vi "NET control example with SP and WFM channels.vi"(8 "error in (no error)":errorcluster, 11 "Node Ptr":T1 format="%.0x") -> (0 "error out":errorcluster)   [LabVIEW 2015]
uses:
  <vilib>/NI Veristand/Custom Device API/Custom Device Item Ref.ctl
  NationalInstruments.VeriStand.SystemStorageUI
  NationalInstruments.VeriStand.SystemStorage
  <vilib>/NI Veristand/Custom Device API/Get Item Property (Dependent Node Pointer).vi
  Shared/Globals/Global GUIDs.vi
  <vilib>/NI Veristand/Custom Device Tools/Custom Device Utility Library/NI VeriStand - Search for All Items by GUID.vi
  <vilib>/NI Veristand/Custom Device API/Set Item Property (Dependent Node Pointer).vi
  <vilib>/NI VeriStand/Custom Device API/Custom Device API.lvlib
  System Explorer/Waveform Data Logger System Explorer.lvlib
  <vilib>/NI VeriStand/Custom Device Tools/Custom Device Utility Library/Custom Device Utility Library.lvlib
  Shared/Waveform Data Logger Shared.lvlib
  <vilib>/NI VeriStand/UI Controls/Single Node Browser/NI_VS UI Single Node Browser.lvlib
panel:
  out ".not. x?":bool
  in  "Source Waveform":refnum<k24>(container)
  in  "Header 2":cluster{"Section Name":string}={"Section Name"="TDMS Data Log Files"}
  in  "Remove":bool
  in  "TDMS Log Files":i32(listbox)
  in  "Add File":bool
  in  "Header":cluster{"Section Name":string}={"Section Name"="Waveform Data Logger Settings"}
  in  "Name":string
  # "TODO: Waveform queue size (auto 3x # wfms, or manual)"
  # "TODO: Mode: one log at a time, one active trigger per log, or log every trigger\n-don't do this. instead using logging group, and allow multiple concurrent triggers for logs with stop trig of \"Duration\""
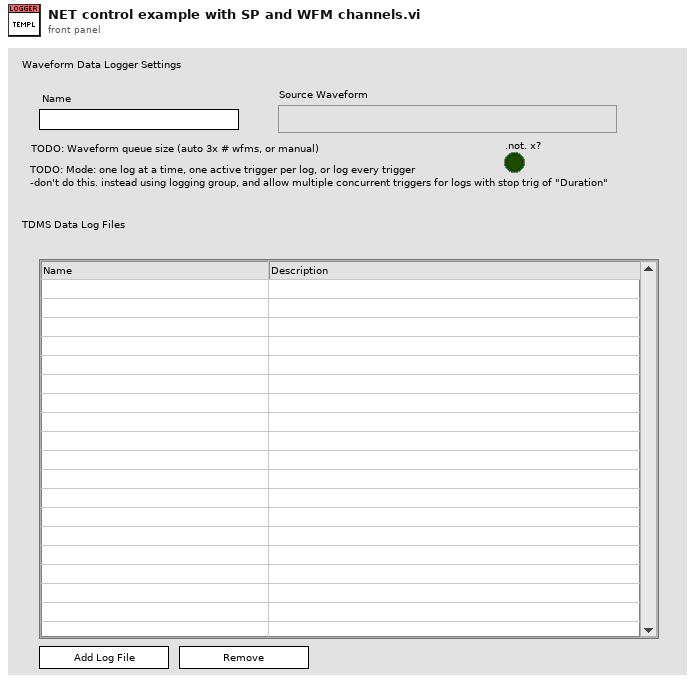
[diagram p1: front panel]
types:
  T1 = typedef "Custom Device API.lvlib/Custom Device Item Ref.ctl" = u64
  T2 = typedef "Custom Device API.lvlib/Custom Device Item Info.ctl" = cluster{"Name":string, "Is Channel":bool, "GUID":string, "Is Waveform":bool}
  T3 = typedef "Custom Device API.lvlib/Custom Device Pointer.ctl" = refnum<k24>
  T4 = typedef "NI_VS UI Single Node Browser.lvlib/Callback Type.ctl" = cluster{"Net Callbacks":refnum<k27>[], "Event":refnum<user-event>}
  T5 = typedef "Custom Device API.lvlib/Custom Device Commands.ctl" = enum16{"Default", "Item renamed", "Shutdown", "Dynamic button pressed"}
  T6 = typedef "LVRowAndColumnTypeDef.ctl" = cluster{"Row":i32, "Column":i32}
  T7 = typedef "NI_VS UI Single Node Browser.lvlib/Node Ref.ctl" = refnum<k24>
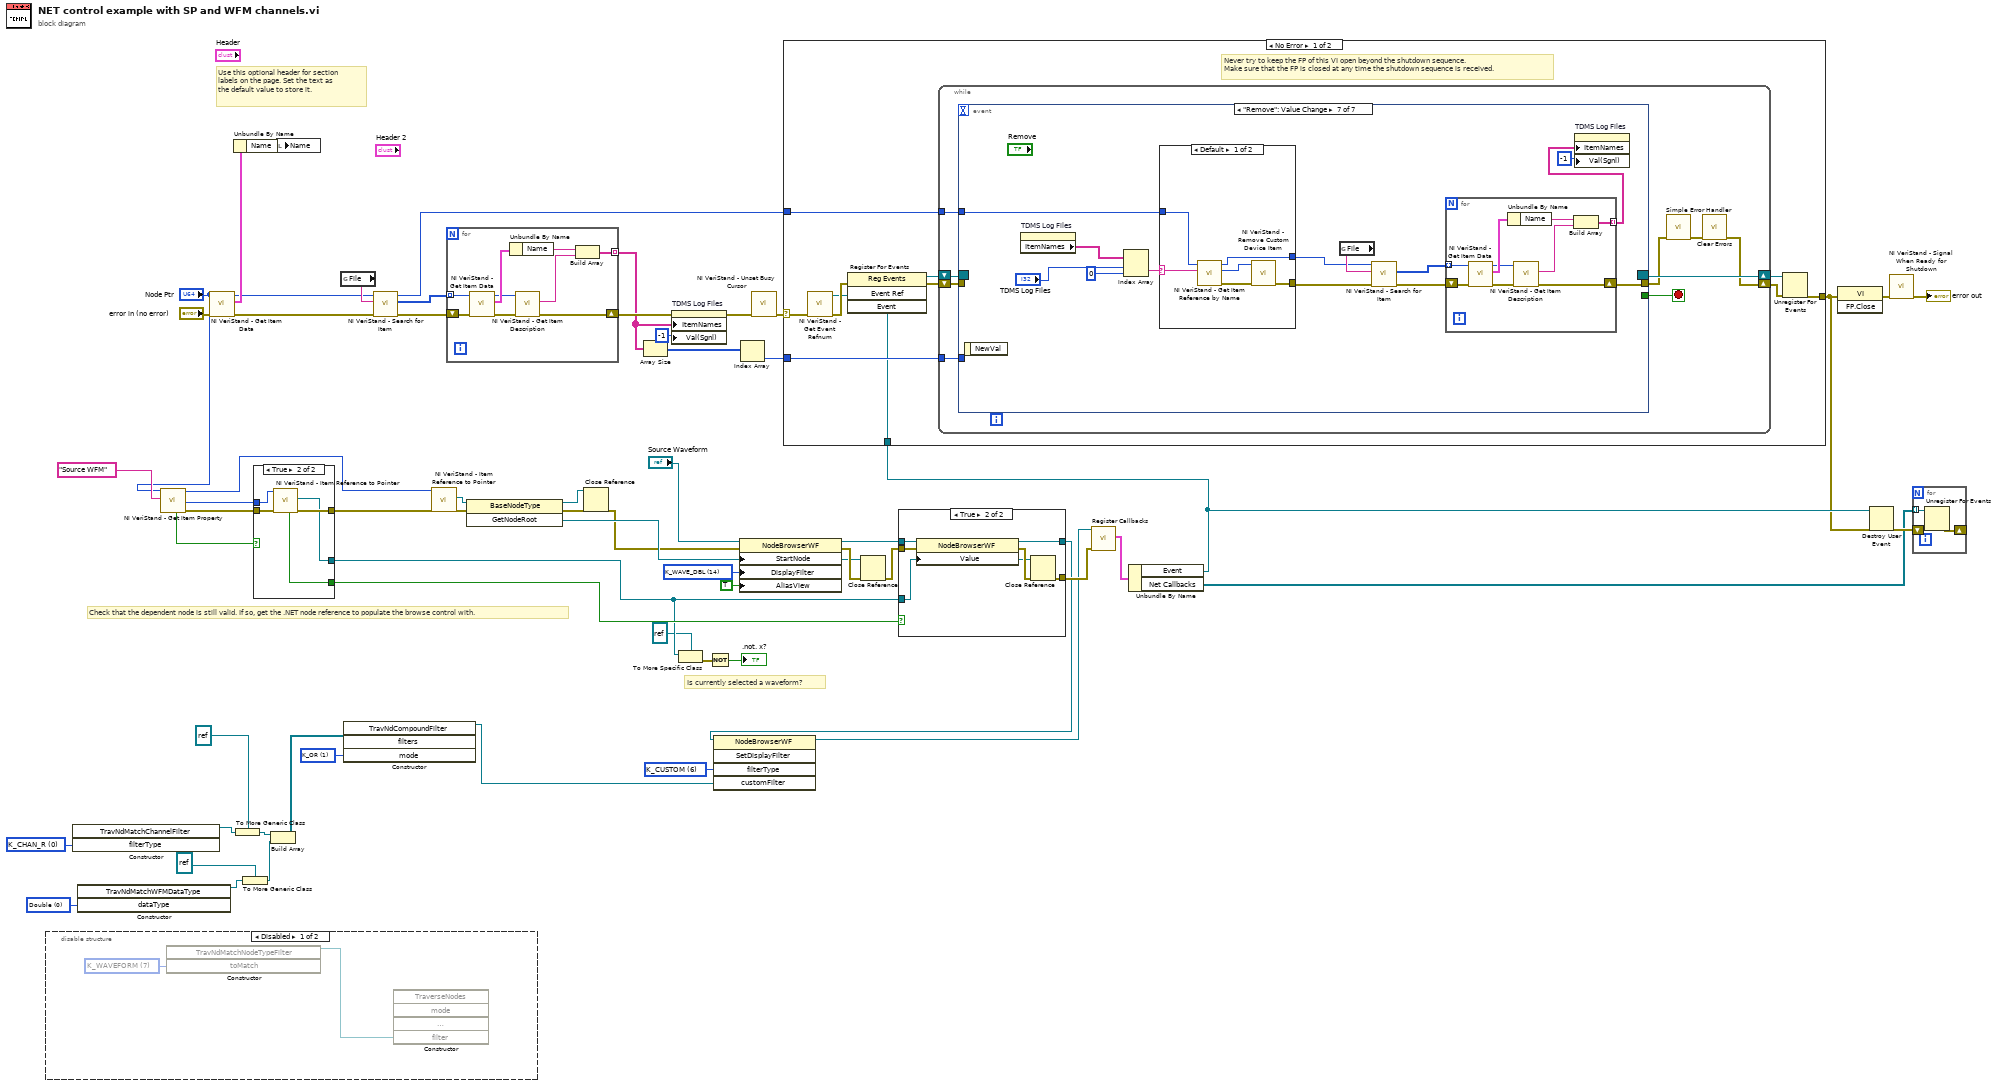
[diagram p0: block diagram]
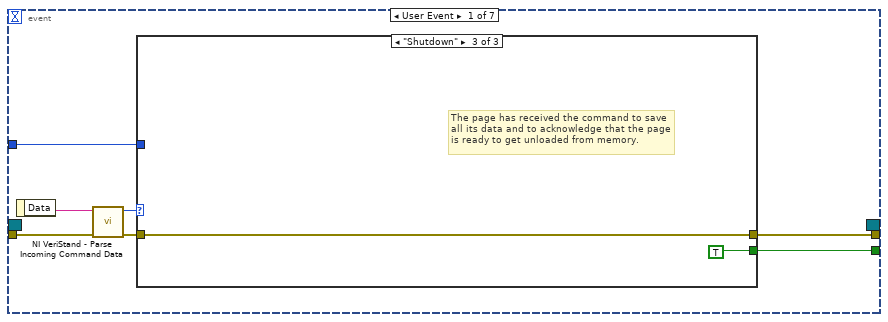
[diagram p5: hidden frame]
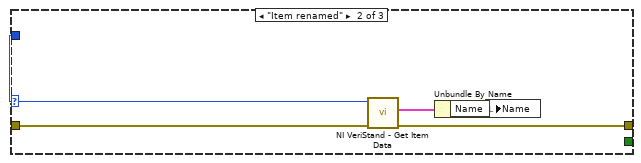
[diagram p7: hidden frame]
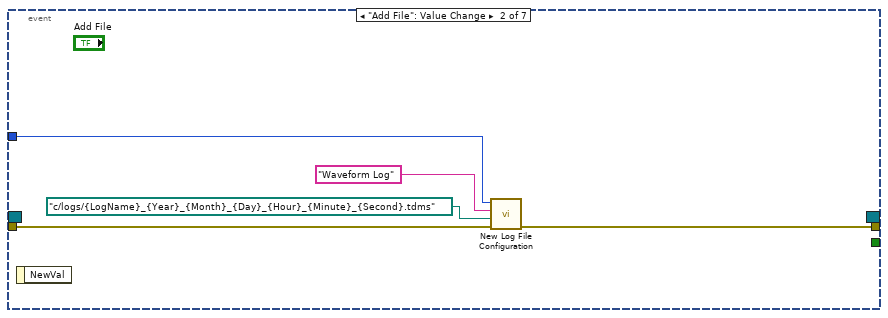
[diagram p8: hidden frame]
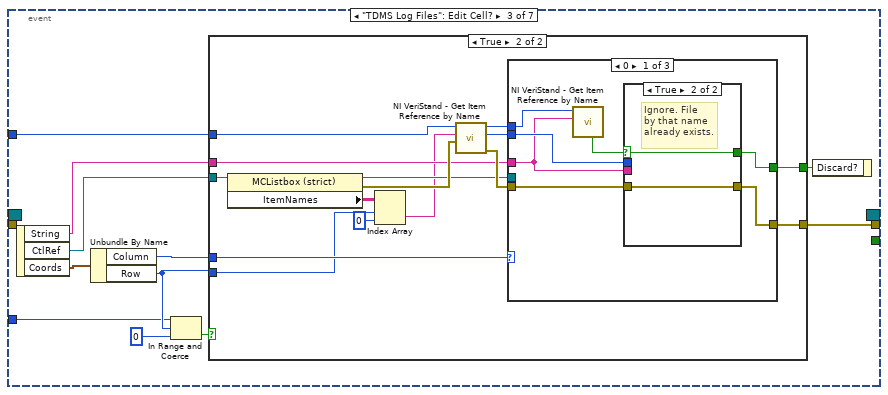
[diagram p9: hidden frame]
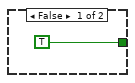
[diagram p10: hidden frame]
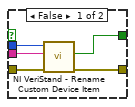
[diagram p11: hidden frame]
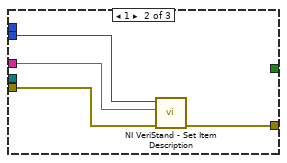
[diagram p12: hidden frame]
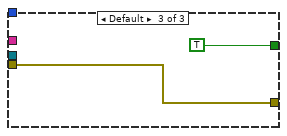
[diagram p13: hidden frame]
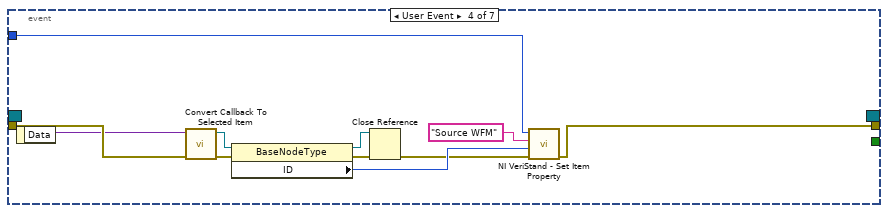
[diagram p14: hidden frame]
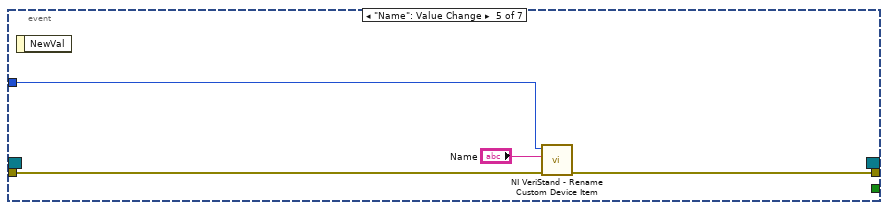
[diagram p15: hidden frame]
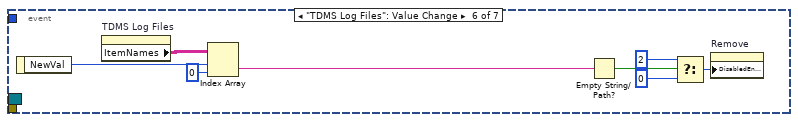
[diagram p16: hidden frame]
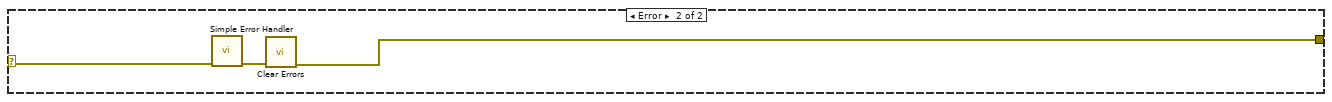
[diagram p18: hidden frame]
diagram:
  w13 = 1 items=["K_AND", "K_OR"] ("mode")
  w14 = 0 items=["Double", "ComplexDouble"] ("dataType")
  w15 = u8 0 items=["K_CHAN_R", "K_CHAN_W", "K_CHAN_VOLT", "K_CHAN_FAULT"] ("filterType")
  w18 = u8 6 items=["K_CHAN_R", "K_CHAN_W", "K_CHAN_RW", "K_CHAN_VOLT", "K_CHAN_FAULT", "K_ALL", "K_CUSTOM", "K_CHAN_R_VIS", "K_CHAN_W_VIS", "K_CHAN_RW_VIS", "K_CHAN_VOLT_VIS", "K_CHAN_FAULT_VIS", "K_WAVE", "K_WAVE_VIS", "K_WAVE_DBL", "K_WAVE_CDB", "K_WAVE_DBL_VIS", "K_WAVE_CDB_VIS"] ("filterType")
  w28 = u8 14 items=["K_CHAN_R", "K_CHAN_W", "K_CHAN_RW", "K_CHAN_VOLT", "K_CHAN_FAULT", "K_ALL", "K_CUSTOM", "K_CHAN_R_VIS", "K_CHAN_W_VIS", "K_CHAN_RW_VIS", "K_CHAN_VOLT_VIS", "K_CHAN_FAULT_VIS", "K_WAVE", "K_WAVE_VIS", "K_WAVE_DBL", "K_WAVE_CDB", "K_WAVE_DBL_VIS", "K_WAVE_CDB_VIS"] ("DisplayFilter")
  # "Is currently selected a waveform?"
  # "Check that the dependent node is still valid. If so, get the .NET node reference to populate the browse control with."
  # "Use this optional header for section labels on the page. Set the text as the default value to store it."
  n1 = disable-structure shown="Disabled" {
    frame Disabled {
      w64 = 7 items=["K_BASE", "K_ALIAS", "K_CHANNEL", "K_SECTION", "K_TARGET", "K_TARGETSECTION", "K_ROOT", "K_WAVEFORM"] ("toMatch")
      n2 = constructor class="TravNdMatchNodeTypeFilter"("toMatch"=w64) -> (reference out=w63:refnum<k24>)  [unwired: 3 in, 3 out]
      n3 = constructor class="TraverseNodes"("filter"=w63) -> ()  [unwired: 5 in, 6 out]
    }
    frame Enabled {
    }
  }
  n4 = constructor class="TravNdMatchChannelFilter"("filterType"=w15) -> (reference out=w12:refnum<k24>)  [unwired: 3 in, 3 out]
  n5 = constructor class="TravNdMatchWFMDataType"("dataType"=w14) -> (reference out=w8:refnum<k24>)  [unwired: 3 in, 3 out]
  n6 = call-poly <vilib>:"NI VeriStand - Get Item Property.vi"("Property Name"="Source WFM", "Item Ref in"="Node Ptr") -> ("error out"=w42:errorcluster, "Dependent Node Ref"=w43:T1, "Item Ref out"=w34:T1, "Found"=w44:bool)  [unwired: 6 in]
  n7 = call <vilib>:"NI VeriStand - Get Item Data.vi"("error in (no error)"="error in (no error)", "Item Ref in"="Node Ptr") -> ("error out"=w45:errorcluster, "Item Info"=w59:T2, "Item Ref out"=w46:T1)  [unwired: 7 out]
  n8 = Unbundle By Name(w59) -> ("Name"=w58:string)
  n9 = To More Generic Class(target class=refnum<k24> refnum, reference=w12) -> (generic class reference=w11:refnum<k24>)
  n10 = To More Generic Class(target class=refnum<k24> refnum, reference=w8) -> (generic class reference=w7:refnum<k24>)
  n11 = case shown="True" w44 {
    selector: w44 -> [w65 _]
    tunnel: [w66 w71] -> w35
    tunnel: [_ w70] -> w4
    tunnel: w42 -> [w66 w69]
    tunnel: w43 -> [_ w68]
    tunnel: [w65 w67] -> w21
    frame False {
    }
    frame True {
      n12 = call <vilib>:"NI VeriStand - Item Reference to Pointer.vi"("error in (no error)"=w69, "Item Ref in"=w68) -> ("error out"=w71:errorcluster, "Node Pointer"=w70:T3, "Found"=w67:bool)  [unwired: 6 in, 1 out]
    }
  }
  n13 = Build Array(w11, w7) -> (w6:refnum<k24>[])
  n14 = local write "Name"(w58) -> ()
  n15 = global read "Global GUIDs.vi" "File"() -> (w47:string)
  n16 = constructor class="TravNdCompoundFilter"("filters"=w6, "mode"=w13) -> (reference out=w5:refnum<k24>)  [unwired: 3 in, 4 out]
  n17 = call-poly <vilib>:"NI VeriStand - Search for Item.vi"("error in"=w45, "Item GUID"=w47, "Section Ref in"=w46) -> ("error out"=w51:errorcluster, "Item Refs"=w50:T1[], "Section Ref out"=w49:T1)  [unwired: 5 in, 1 out]
  n18 = call <vilib>:"NI VeriStand - Item Reference to Pointer.vi"("error in (no error)"=w35, "Item Ref in"=w34) -> ("error out"=w38:errorcluster, "Node Pointer"=w37:T3)  [unwired: 6 in, 2 out]
  n19 = for {
    tunnel: w50 -> [w79] mode=indexing
    tunnel: [w75] -> w54 mode=indexing
    shift-right: [w74] -> w57
    shift-left: w51 -> [w80]
    n20 = call <vilib>:"NI VeriStand - Get Item Data.vi"("error in (no error)"=w80, "Item Ref in"=w79) -> ("error out"=w72:errorcluster, "Item Info"=w78:T2, "Item Ref out"=w73:T1)  [unwired: 6 in, 1 out]
    n21 = Unbundle By Name(w78) -> ("Name"=w77:string)
    n22 = call <vilib>:"NI VeriStand - Get Item Description.vi"("error in (no error)"=w72, "Item Ref in"=w73) -> ("error out"=w74:errorcluster, "Description"=w76:string)  [unwired: 6 in, 2 out]
    n23 = Build Array(w77, w76) -> (w75:string[])
  }
  n24 = invoke class="BaseNodeType" method="GetNodeRoot"(reference=w37, error in=w38) -> (reference out=w40:T3, error out=w39:errorcluster, "GetNodeRoot"=w22:refnum<k24>)  [unwired: 1 in]
  n25 = Close Reference(reference=w40, error in (no error)=w39) -> (error out=w20:errorcluster)
  n26 = Array Size(array=w54) -> (size(s)=w53:i32[])
  n27 = property on="TDMS Log Files" class="MCListbox (strict)"(error in=w57, "ItemNames"=w54, "Val(Sgnl)"=-1 ("Value (Signaling)")) -> (error out=w55:errorcluster)  [unwired: 1 in, 1 out]
  n28 = To More Specific Class(target class=refnum<k24> refnum, reference=w4) -> (error out=w1:errorcluster)  [unwired: 1 in, 1 out]
  n29 = Not(x=w1) -> (.not. x?=→".not. x?":bool)
  n30 = property class="NodeBrowserWF"(reference="Source Waveform", error in=w20, "StartNode"=w22, "DisplayFilter"=w28, "AliasView"=TRUE) -> (reference out=w33:refnum<k24>, error out=w30:errorcluster)
  n31 = Index Array(array=w53) -> (element=w52:i32)  [unwired: 1 in]
  n32 = call <vilib>:"NI VeriStand - Unset Busy Cursor.vi"("error in (no error)"=w55) -> ("error out"=w60:errorcluster)  [unwired: 10 out]
  n33 = Close Reference(reference=w22, error in (no error)=w30) -> (error out=w32:errorcluster)
  n34 = case shown="True" w21 {
    tunnel: [w81 w88] -> w31
    tunnel: w32 -> [w81 w87]
    tunnel: w33 -> [w82 w86]
    tunnel: [w82 w84] -> w17
    tunnel: w4 -> [_ w83]
    frame False {
    }
    frame True {
      n35 = property class="NodeBrowserWF"(reference=w86, error in=w87, "Value"=w83) -> (reference out=w84:refnum<k24>, error out=w85:errorcluster)
      n36 = Close Reference(reference=w83, error in (no error)=w85) -> (error out=w88:errorcluster)
    }
  }
  n37 = invoke class="NodeBrowserWF" method="SetDisplayFilter"(reference=w17, "filterType"=w18, "customFilter"=w5) -> (reference out=w16:refnum<k24>)  [unwired: 2 in, 4 out]
  n38 = call <vilib>:"Register Callbacks.vi"("error in (no error)"=w31, "Single Node Browser"=w16) -> ("Callbacks"=w27:T4)  [unwired: 7 in, 2 out]
  n39 = Unbundle By Name(w27) -> ("Event"=w25:refnum<user-event>, "Net Callbacks"=w24:refnum<k27>[])
  n40 = case shown="No Error" w60 {
    selector: w60 -> [w91 w230]
    tunnel: [w96 w228] -> w23
    tunnel: w49 -> [w92 _]
    tunnel: w52 -> [w90 _]
    tunnel: w25 -> [w89 _]
    frame No Error {
      # "Never try to keep the FP of this VI open beyond the shutdown sequence.\nMake sure that the FP is closed at any time the shutdown sequence is received."
      n41 = call <vilib>:"NI VeriStand - Get Event Refnum.vi"("error in (no error)"=w91) -> ("error out"=w99:errorcluster, "Event Ref"=w95:refnum<user-event>)  [unwired: 9 out]
      n42 = register-events(error in=w99, w95, w89) -> (reference out=w93:refnum<event-registration>, error out=w94:errorcluster)  [unwired: 1 in]
      n43 = while {
        tunnel: w92 -> [w104]
        shift-right: [w101] -> w97
        shift-left: w94 -> [w107]
        shift-right: [w108] -> w98
        shift-left: w93 -> [w106]
        tunnel: w90 -> [w100]
        stop <- w105 stop-if-true
        n44 = event shown="[6] \"Remove\": Value Change" {
          selector: w106 -> [_ _ _ _ _ _ _]
          dyn-events: [_ _ _ _ _ _ _] -> w108
          timeout: _ -> [_ _ _ _ _ _ _]
          tunnel: w107 -> [w115 w127 _ w179 w190 _ _]
          tunnel: [w111 _ _ _ _ _ _] -> w105
          tunnel: [w110 w126 w135 w176 w189 _ w201] -> w103
          tunnel: w104 -> [w109 w128 w130 w177 w188 _ w209]
          tunnel: w100 -> [_ _ w129 _ _ _ _]
          event User Event {
            n45 = event-data() -> ("Data"=w114:string)  [unwired: 1 out]
            n46 = call <vilib>:"NI VeriStand - Parse Incoming Command Data.vi"("error in (no error)"=w115, "Incoming data"=w114) -> ("error out"=w113:errorcluster, "Action"=w112:T5)  [unwired: 8 out]
            n47 = case shown="\"Shutdown\"" w112 {
              tunnel: w113 -> [w116 w121 w122]
              tunnel: [_ _ TRUE] -> w111
              tunnel: [w116 w118 w122] -> w110
              tunnel: w109 -> [_ w120 _]
              frame "Default", Default {
              }
              frame "Item renamed" {
                n48 = call <vilib>:"NI VeriStand - Get Item Data.vi"("error in (no error)"=w121, "Item Ref in"=w120) -> ("error out"=w118:errorcluster, "Item Info"=w119:T2)  [unwired: 8 out]
                n49 = Unbundle By Name(w119) -> ("Name"=w117:string)
                n50 = local write "Name"(w117) -> ()
              }
              frame "Shutdown" {
                # "The page has received the command to save all its data and to acknowledge that the page is ready to get unloaded from memory."
              }
            }
          }
          event "Add File": Value Change {
            n51 = event-data() -> ()  [unwired: 2 out]
            n52 = call "New Log File Configuration.vi"("error in (no error)"=w127, "Default Path"=path "c:/logs/{LogName}_{Year}_{Month}_{Day}_{Hour}_{Minute}_{Second}.tdms" ("Default Log Directory"), "Default Name"="Waveform Log", "Device Ref in"=w128) -> ("error out"=w126:errorcluster)  [unwired: 7 out]
          }
          event "TDMS Log Files": Edit Cell? {
            n53 = event-data() -> ("String"=w132:string, "CtlRef"=w131:refnum<vi>, "Coords"=w133:T6)  [unwired: 1 out]
            n54 = Unbundle By Name(w133) -> ("Column"=w139:i32, "Row"=w137:i32)
            n55 = In Range and Coerce(upper limit=w129, x=w137, lower limit=0) -> (In Range?=w136:bool)  [unwired: 1 out]
            n56 = case shown="True" w136 {
              tunnel: w131 -> [_ w153]
              tunnel: [TRUE w150] -> w134
              tunnel: w132 -> [_ w148]
              tunnel: w130 -> [_ w146]
              tunnel: w137 -> [_ w145]
              tunnel: w139 -> [_ w151]
              tunnel: [_ w147] -> w135
              frame False {
              }
              frame True {
                n57 = property class="MCListbox (strict)"(reference=w153) -> (reference out=w149:refnum<vi>, error out=w155:errorcluster, "ItemNames"=w152:string[][])  [unwired: 1 in]
                n58 = Index Array(array=w152, index (row)=w145, index (col)=0 ("disabled index (col)")) -> (element=w143:string)
                n59 = call <vilib>:"NI VeriStand - Get Item Reference by Name.vi"("error in (no error)"=w155, "Item Name"=w143, "Parent Ref in"=w146) -> ("error out"=w154:errorcluster, "Item Ref"=w142:T1, "Parent Ref out"=w141:T1)  [unwired: 5 in, 1 out]
                n60 = case shown="0" w151 {
                  tunnel: [w156 _ TRUE] -> w150
                  tunnel: w142 -> [w161 w172 _]
                  tunnel: w154 -> [w162 w170 w174]
                  tunnel: w149 -> [_ _ _]
                  tunnel: w148 -> [w158 w171 _]
                  tunnel: [w160 w173 w174] -> w147
                  tunnel: w141 -> [w159 _ _]
                  frame 0 {
                    n61 = call <vilib>:"NI VeriStand - Get Item Reference by Name.vi"("Item Name"=w158, "Parent Ref in"=w159) -> ("Found"=w157:bool)  [unwired: 6 in, 3 out]
                    n62 = case shown="True" w157 {
                      selector: w157 -> [_ w168]
                      tunnel: w162 -> [w167 w169]
                      tunnel: w161 -> [w166 _]
                      tunnel: [w165 w169] -> w160
                      tunnel: w158 -> [w164 _]
                      tunnel: [w163 w168] -> w156
                      frame False {
                        n63 = call <vilib>:"NI VeriStand - Rename Custom Device Item.vi"("error in (no error)"=w167, "New Name"=w164, "Item Ref in"=w166) -> ("error out"=w165:errorcluster, "Request invalid?"=w163:bool)  [unwired: 6 in, 1 out]
                      }
                      frame True {
                        # "Ignore. File\nby that name\nalready exists."
                      }
                    }
                  }
                  frame 1 {
                    n64 = call <vilib>:"NI VeriStand - Set Item Description.vi"("error in (no error)"=w170, "Description"=w171, "Item Ref in"=w172) -> ("error out"=w173:errorcluster)  [unwired: 6 in, 2 out]
                  }
                  frame Default {
                  }
                }
              }
            }
            n65 = event-data("Discard?"=w134) -> ()  [unwired: 1 in, 1 out]
          }
          event User Event {
            n66 = event-data() -> ("Data"=w178:variant)  [unwired: 1 out]
            n67 = call <vilib>:"Convert Callback To Selected Item.vi"("error in"=w179, "Data"=w178) -> ("error out"=w180:errorcluster, "Selected Item"=w181:T7)  [unwired: 8 in]
            n68 = property class="BaseNodeType"(reference=w181, error in=w180) -> (reference out=w183:T7, error out=w182:errorcluster, "ID"=w186:u64)
            n69 = Close Reference(reference=w183, error in (no error)=w182) -> (error out=w185:errorcluster)
            n70 = call-poly <vilib>:"NI VeriStand - Set Item Property.vi"("error in (no error)"=w185, "Dependent Node Ref"=w186, "Property Name"="Source WFM", "Item Ref in"=w177) -> ("error out"=w176:errorcluster)  [unwired: 5 in, 2 out]
          }
          event "Name": Value Change {
            n71 = event-data() -> ()  [unwired: 2 out]
            n72 = call <vilib>:"NI VeriStand - Rename Custom Device Item.vi"("error in (no error)"=w190, "New Name"="Name", "Item Ref in"=w188) -> ("error out"=w189:errorcluster)  [unwired: 1 in, 7 out]
          }
          event "TDMS Log Files": Value Change {
            n73 = event-data() -> ("NewVal"=w191:i32)  [unwired: 1 out]
            n74 = property on="TDMS Log Files" class="MCListbox (strict)"() -> ("ItemNames"=w192:string[][])  [unwired: 2 in, 2 out]
            n75 = Index Array(array=w192, index (row)=w191, index (col)=0 ("disabled index (col)")) -> (element=w195:string)
            n76 = Empty String/Path?(string/path=w195) -> (empty?=w194:bool)
            n77 = Select(t=u8 2, s=w194, f=u8 0) -> (s? t:f=w196:u8)
            n78 = property on="Remove" class="Bool"("DisabledEnum"=w196) -> ()  [unwired: 2 in, 2 out]
          }
          event "Remove": Value Change {
            n79 = event-data() -> ()  [unwired: 2 out]
            n80 = property on="TDMS Log Files" class="MCListbox (strict)"() -> ("ItemNames"=w208:string[][])  [unwired: 2 in, 2 out]
            n81 = Index Array(array=w208, index (row)="TDMS Log Files", index (col)=0 ("disabled index (col)")) -> (element=w211:string)
            n82 = case shown="Default" w211 {
              selector: w211 -> [w223 _]
              tunnel: w209 -> [w224 w227]
              tunnel: [w226 _] -> w200
              tunnel: [w221 w227] -> w199
              frame Default {
                n83 = call <vilib>:"NI VeriStand - Get Item Reference by Name.vi"("Item Name"=w223, "Parent Ref in"=w224) -> ("error out"=w225:errorcluster, "Item Ref"=w222:T1, "Parent Ref out"=w221:T1)  [unwired: 6 in, 1 out]
                n84 = call <vilib>:"NI VeriStand - Remove Custom Device Item.vi"("error in (no error)"=w225, "Item Ref in"=w222) -> ("error out"=w226:errorcluster)  [unwired: 8 in, 1 out]
              }
              frame "" {
              }
            }
            n85 = global read "Global GUIDs.vi" "File"() -> (w204:string)
            n86 = call-poly <vilib>:"NI VeriStand - Search for Item.vi"("error in"=w200, "Item GUID"=w204, "Section Ref in"=w199) -> ("error out"=w206:errorcluster, "Item Refs"=w205:T1[])  [unwired: 5 in, 2 out]
            n87 = for {
              tunnel: w205 -> [w219] mode=indexing
              tunnel: [w215] -> w202 mode=indexing
              shift-right: [w214] -> w201
              shift-left: w206 -> [w220]
              n88 = call <vilib>:"NI VeriStand - Get Item Data.vi"("error in (no error)"=w220, "Item Ref in"=w219) -> ("error out"=w212:errorcluster, "Item Info"=w218:T2, "Item Ref out"=w213:T1)  [unwired: 6 in, 1 out]
              n89 = Unbundle By Name(w218) -> ("Name"=w217:string)
              n90 = call <vilib>:"NI VeriStand - Get Item Description.vi"("error in (no error)"=w212, "Item Ref in"=w213) -> ("error out"=w214:errorcluster, "Description"=w216:string)  [unwired: 6 in, 2 out]
              n91 = Build Array(w217, w216) -> (w215:string[])
            }
            n92 = property on="TDMS Log Files" class="MCListbox (strict)"("ItemNames"=w202, "Val(Sgnl)"=-1 ("Value (Signaling)")) -> ()  [unwired: 2 in, 2 out]
          }
        }
        n93 = call <vilib>:"Simple Error Handler.vi"("error in (no error)"=w103) -> ("error out"=w102:errorcluster)  [unwired: 1 in, 7 out]
        n94 = call <vilib>:"Clear Errors.vi"("error in (no error)"=w102) -> ("error out"=w101:errorcluster)  [unwired: 1 in, 5 out]
      }
      n95 = Unregister For Events(event registration refnum=w98, error in=w97) -> (error out=w96:errorcluster)
    }
    frame Error {
      n96 = call <vilib>:"Simple Error Handler.vi"("error in (no error)"=w230) -> ("error out"=w229:errorcluster)  [unwired: 1 in, 7 out]
      n97 = call <vilib>:"Clear Errors.vi"("error in (no error)"=w229) -> ("error out"=w228:errorcluster)  [unwired: 1 in, 5 out]
    }
  }
  n98 = invoke class="VI" method="FP.Close"(error in=w23) -> (error out=w62:errorcluster)  [unwired: 2 in, 2 out]
  n99 = Destroy User Event(user event=w25, error in=w23) -> (error out=w26:errorcluster)
  n100 = call <vilib>:"NI VeriStand - Signal When Ready for Shutdown.vi"("error in (no error)"=w62) -> ("error out"=→"error out":errorcluster)  [unwired: 10 out]
  n101 = for {
    tunnel: w24 -> [w231] mode=indexing
    shift-right: [w232] -> _
    shift-left: w26 -> [w233]
    n102 = Unregister For Events(event registration refnum=w231, error in=w233) -> (error out=w232:errorcluster)
  }
